vi "USBImageWthFileOutputManual.vi"() -> ()   [LabVIEW 2017]
uses:
  <vilib>/Utility/file.llb/Write Delimited Spreadsheet (I64).vi
  atmcd32d.dll
panel:
  in  "?":bool
  in  "?":bool
  out "Status":u32
  out "Get Status":u32
  out "Vertical Binned Waveform Graph":i32[](graph)
  out "Intensity Graph":i32[][](graph)
  out "Set Image":u32
  out "Set Gate Mode":u32
  out "Shut Down":u32
  out "Detector Y Pixels":i32
  out "Get Detector":u32
  out "Set Exposure Time":u32
  out "Set Trigger Mode":u32
  out "Set Readout Mode":u32
  out "Set Acquisition Mode":u32
  out "Check Timings":u32
  out "Detector X Pixels":i32
  out "Start Acquisition":u32
  out "Get Acquired Data":u32
  out "Calculated Exposure Value":sgl format="%.5f"
  in  "Exposure Time (secs)":sgl format="%.2f"
  out "Initialize":u32
  in  "Trigger":u32(ring) items=["Internal", "External"]
  # "Status"
  # "Return values"
  # "USB iStarIMAG32at.VI"
  # "Acquisition Mode: Single Scan\nReadout Mode: Full Resolution Image"
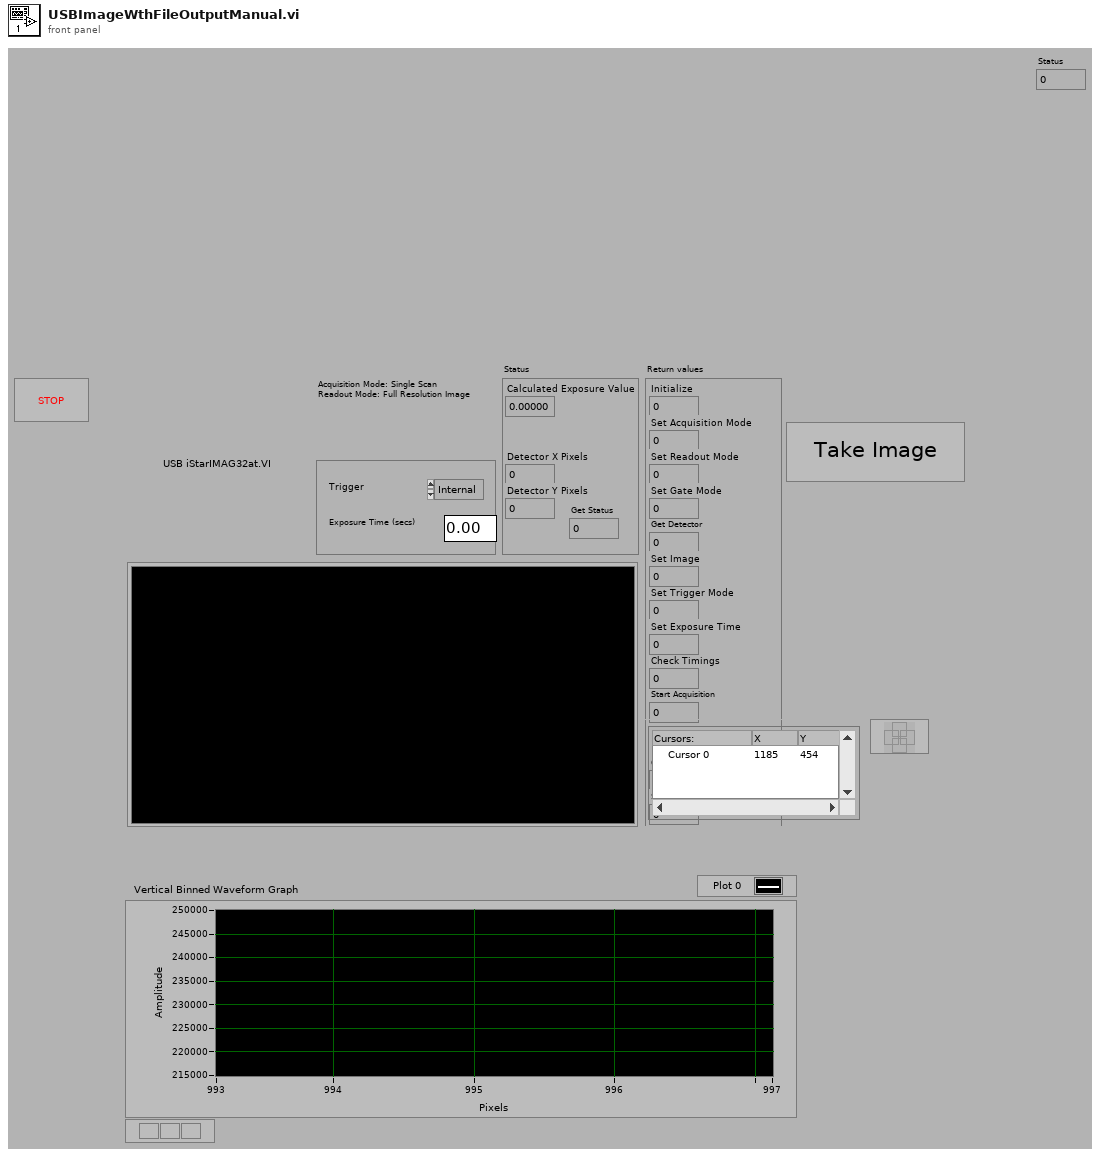
[diagram p1: front panel]
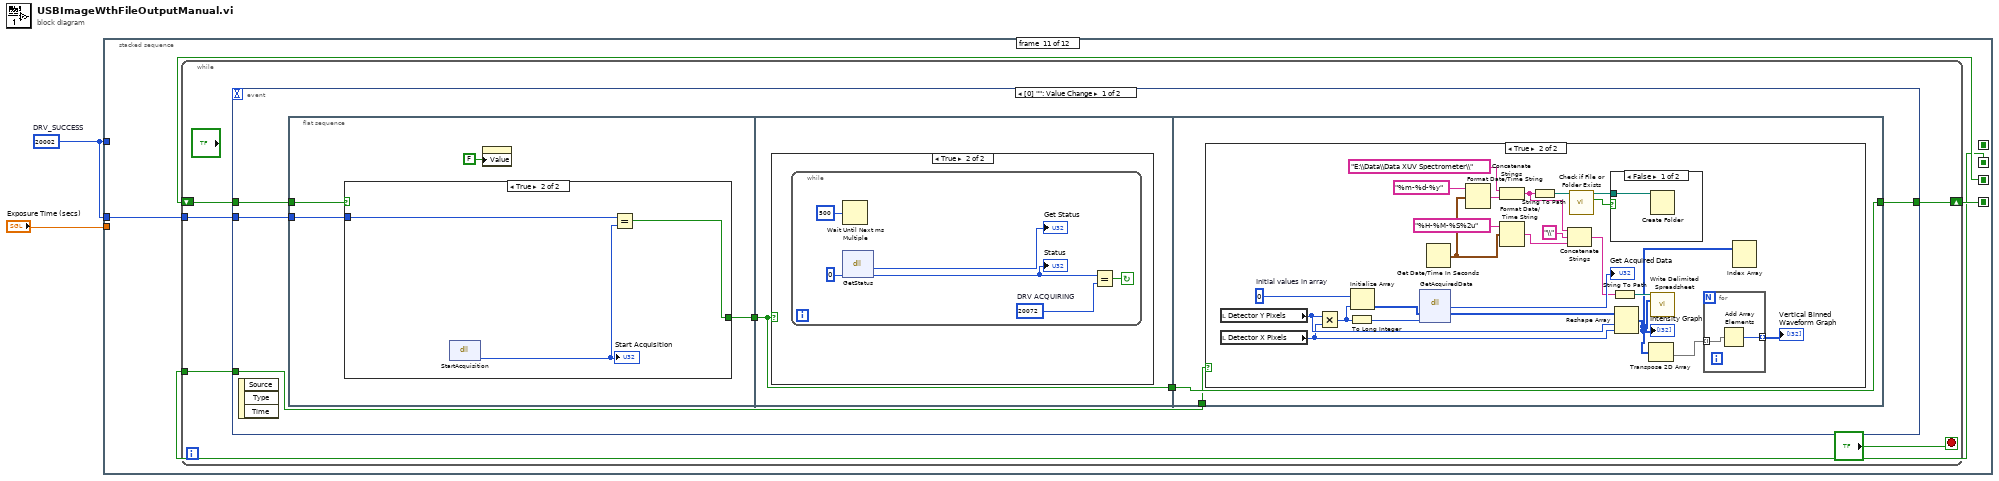
[diagram p0: block diagram]
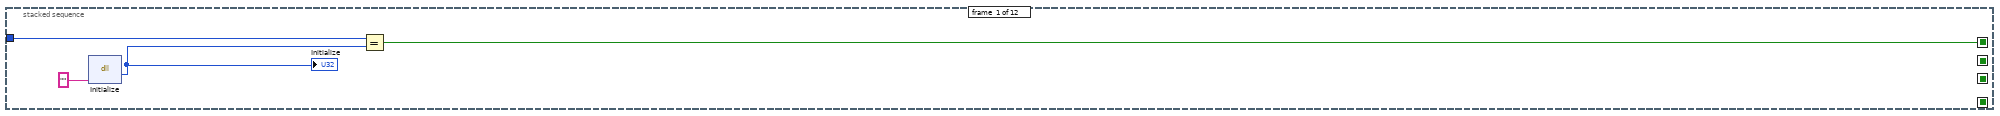
[diagram p2: hidden frame]
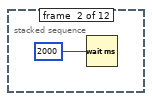
[diagram p3: hidden frame]
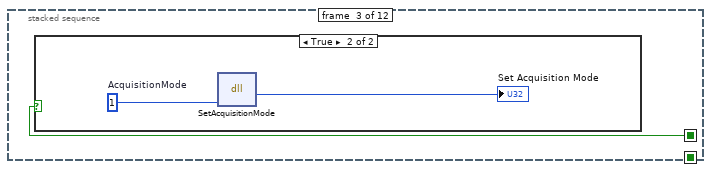
[diagram p4: hidden frame]
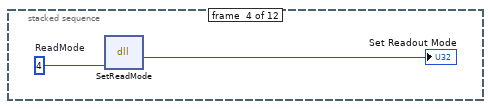
[diagram p6: hidden frame]
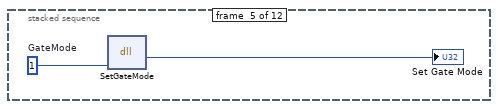
[diagram p7: hidden frame]
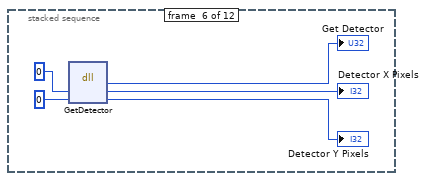
[diagram p8: hidden frame]
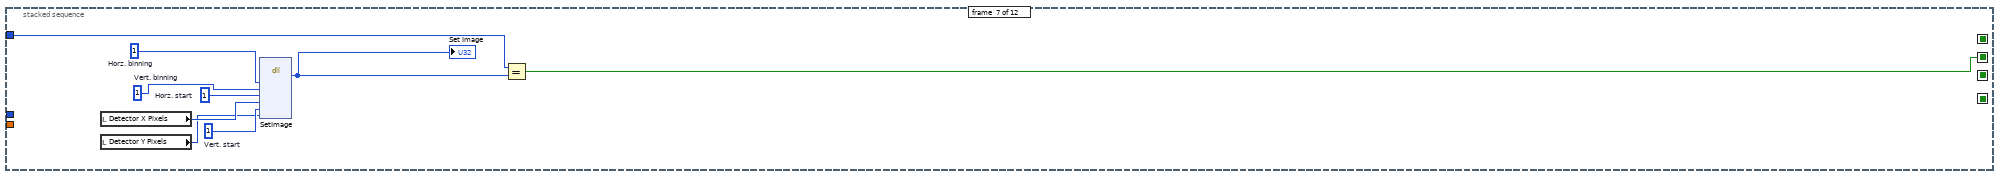
[diagram p9: hidden frame]
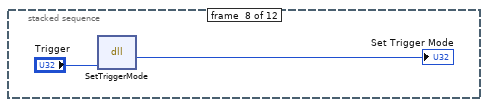
[diagram p10: hidden frame]
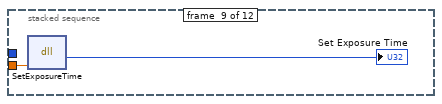
[diagram p11: hidden frame]
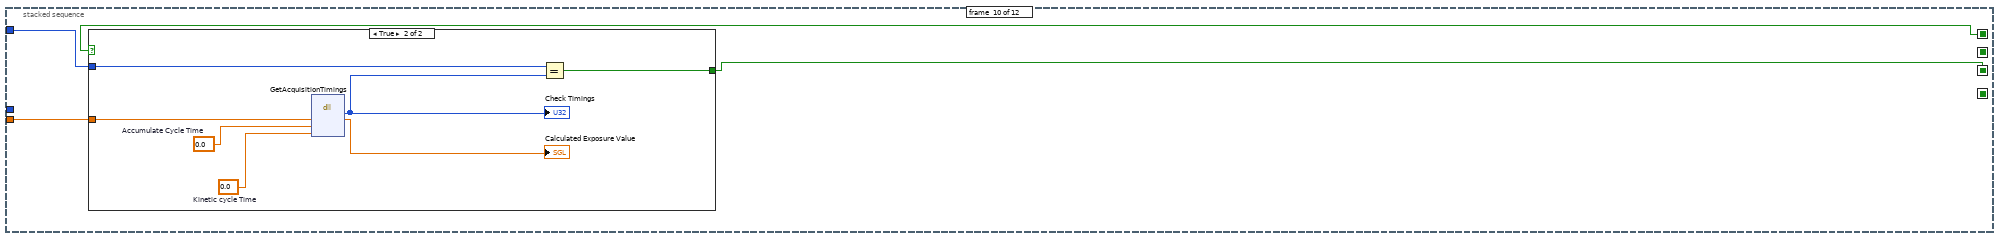
[diagram p12: hidden frame]
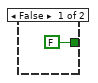
[diagram p13: hidden frame]
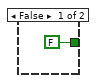
[diagram p14: hidden frame]
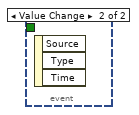
[diagram p18: hidden frame]
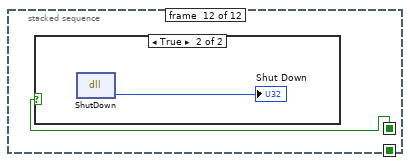
[diagram p19: hidden frame]
diagram:
  w1 = 20002  # DRV_SUCCESS
  n1 = stacked-sequence {
    seq-local: [w4 _ _ _ _ _ _ _ _ _ _ _] -> [_ _ w8 _ _ _ _ _ _ w33 _ w104]
    seq-local: [_ _ _ _ _ _ _ _ _ w34 _ _] -> [_ _ _ _ _ _ _ _ _ _ w48 _]
    seq-local: [_ _ _ _ _ _ _ _ _ _ w46 _] -> [_ _ _ _ _ _ _ _ _ _ _ _]
    seq-local: [_ _ _ _ _ _ w20 _ _ _ _ _] -> [_ _ _ _ _ _ _ _ _ _ w45 _]
    tunnel: "Exposure Time (secs)" -> [_ _ _ _ _ _ _ _ w32 w36 _ _]
    tunnel: w1 -> [w5 _ _ _ _ _ w22 _ _ w35 _ _]
    tunnel: w1 -> [_ _ _ _ _ _ _ _ _ _ w47 _]
    frame #0 {
      n2 = dll-call lib="atmcd32d.dll" fn="Initialize" label="Call Library Function Initialize"("") -> (w6:u32)  [unwired: 4 in, 2 out]
      "Initialize" <- w6
      n3 = Equal?(x=w5, y=w6) -> (x = y?=w4:bool)
    }
    frame #1 {
      n4 = Wait (ms)(milliseconds to wait=u32 2000) -> ()  [unwired: 1 out]
    }
    frame #2 {
      n5 = case shown="True" w8 {
        frame False {
        }
        frame True {
          w10 = u16 1  # AcquisitionMode
          n6 = dll-call lib="atmcd32d.dll" fn="SetAcquisitionMode" label="Call Library Function SetAcquisitionMode"(w10) -> (→"Set Acquisition Mode":u32)  [unwired: 4 in, 2 out]
        }
      }
    }
    frame #3 {
      w12 = u16 4  # ReadMode
      n7 = dll-call lib="atmcd32d.dll" fn="SetReadMode" label="Call Library Function SetReadMode"(w12) -> (→"Set Readout Mode":u32)  [unwired: 4 in, 2 out]
    }
    frame #4 {
      w14 = u16 1  # GateMode
      n8 = dll-call lib="atmcd32d.dll" fn="SetGateMode" label="Call Library Function SetGateMode"(w14) -> (→"Set Gate Mode":u32)  [unwired: 4 in, 2 out]
    }
    frame #5 {
      n9 = dll-call lib="atmcd32d.dll" fn="GetDetector" label="Call Library FunctionGetDetector"(i16 0, i16 0) -> (→"Get Detector":u32, →"Detector X Pixels":i32, →"Detector Y Pixels":i32)  [unwired: 3 in, 2 out]
    }
    frame #6 {
      w25 = u16 1  # Vert. start
      w26 = u16 1  # Horz. start
      w27 = u16 1  # Vert. binning
      w28 = u16 1  # Horz. binning
      n10 = local read "Detector X Pixels"() -> (w24:i32)
      n11 = local read "Detector Y Pixels"() -> (w23:i32)
      n12 = dll-call lib="atmcd32d.dll" fn="SetImage" label="Call Library Function SetImage"(w28, w27, w26, w24, w25, w23) -> (w21:u32)  [unwired: 9 in, 2 out]
      "Set Image" <- w21
      n13 = Equal?(x=w22, y=w21) -> (x = y?=w20:bool)
    }
    frame #7 {
      n14 = dll-call lib="atmcd32d.dll" fn="SetTriggerMode" label="Call Library Function SetTrigger Mode"("Trigger") -> (→"Set Trigger Mode":u32)  [unwired: 4 in, 2 out]
    }
    frame #8 {
      n15 = dll-call lib="atmcd32d.dll" fn="SetExposureTime" label="Call Library FunctionSet Exposure Time"(w32) -> (→"Set Exposure Time":u32)  [unwired: 4 in, 2 out]
    }
    frame #9 {
      n16 = case shown="True" w33 {
        tunnel: w36 -> [_ w41]
        tunnel: w35 -> [_ w38]
        tunnel: [FALSE w40] -> w34
        frame False {
        }
        frame True {
          w43 = sgl 0.0  # Accumulate Cycle Time
          w44 = sgl 0.0  # Kinetic cycle Time
          n17 = dll-call lib="atmcd32d.dll" fn="GetAcquisitionTimings" label="Call Library Function Check Timings"(w41, w43, w44) -> (w39:u32, →"Calculated Exposure Value":sgl)  [unwired: 5 in, 2 out]
          "Check Timings" <- w39
          n18 = Equal?(x=w38, y=w39) -> (x = y?=w40:bool)
        }
      }
    }
    frame #10 {
      n19 = while {
        tunnel: w47 -> [w52]
        tunnel: w45 -> [w50]
        shift-right: [w51] -> w46
        shift-left: w48 -> [w53]
        stop <- "?" stop-if-true
        n20 = event shown="[0] \"\": Value Change" {
          selector: _ -> [_ _]
          dyn-events: _ -> [_ _]
          timeout: _ -> [_ _]
          tunnel: w53 -> [w57 _]
          tunnel: w52 -> [w56 _]
          tunnel: [w55 _] -> w51
          tunnel: w50 -> [w54 _]
          event Value Change {
            n21 = event-data() -> ()  [unwired: 1 in, 3 out]
            n22 = flat-sequence {
              tunnel: w57 -> [w63]
              tunnel: w56 -> [w62]
              tunnel: [w61] -> w59
              tunnel: w59 -> [w68]
              tunnel: [w68] -> w58
              tunnel: [w76] -> w55
              tunnel: w58 -> [w76]
              tunnel: w54 -> [w75]
              frame #0 {
                n23 = case shown="True" w63 {
                  tunnel: [FALSE w66] -> w61
                  tunnel: w62 -> [_ w65]
                  frame False {
                  }
                  frame True {
                    n24 = dll-call lib="atmcd32d.dll" fn="StartAcquisition" label="Call Library Function start acquisition"() -> (w67:u32)  [unwired: 3 in, 2 out]
                    "Start Acquisition" <- w67
                    n25 = Equal?(x=w65, y=w67) -> (x = y?=w66:bool)
                  }
                }
                n26 = property class="Bool (strict)"("Value"=FALSE ("Take image")) -> ()  [unwired: 2 in, 2 out]
              }
              frame #1 {
                n27 = case shown="True" w68 {
                  frame False {
                  }
                  frame True {
                    n28 = while {
                      stop <- w72 continue-if-true
                      w71 = u16 20072  # DRV ACQUIRING
                      n29 = Wait Until Next ms Multiple(millisecond multiple=u32 500) -> ()  [unwired: 1 out]
                      n30 = dll-call lib="atmcd32d.dll" fn="GetStatus" label="Call Library Function GetAcquisitionStatus"(u16 0) -> (→"Get Status":u32, w70:u32)  [unwired: 3 in, 2 out]
                      "Status" <- w70
                      n31 = Equal?(x=w70, y=w71) -> (x = y?=w72:bool)
                    }
                  }
                }
              }
              frame #2 {
                n32 = case shown="True" w75 {
                  frame False {
                  }
                  frame True {
                    w100 = 0  # Initial values in array
                    n33 = local read "Detector Y Pixels"() -> (w94:i32)
                    n34 = local read "Detector X Pixels"() -> (w93:i32)
                    n35 = Multiply(x=w94, y=w93) -> (x*y=w96:i32)
                    n36 = To Long Integer(number=w96) -> (32bit integer=w97:i32)
                    n37 = Initialize Array "Initialize Array"(w100, w96) -> (w98:i32[])
                    n38 = dll-call lib="atmcd32d.dll" fn="GetAcquiredData" label="Call Library Function Get Acquired data"(w98, w97) -> (→"Get Acquired Data":u32, w95:i32[])  [unwired: 4 in, 2 out]
                    n39 = Get Date/Time In Seconds() -> (seconds since 1Jan1904=w90:timestamp)
                    n40 = Format Date/Time String(time format string (%c)="%m-%d-%y", seconds (now)=w90) -> (date/time string=w88:string)  [unwired: 1 in]
                    n41 = Concatenate Strings("E:\\Data\\Data XUV Spectrometer\\" ("string"), w88) -> (w91:string)
                    n42 = Format Date/Time String(time format string (%c)="%H-%M-%S%2u", seconds (now)=w90) -> (date/time string=w89:string)  [unwired: 1 in]
                    n43 = String To Path(string=w91) -> (path=w87:path)
                    n44 = Concatenate Strings(w91, "\\" ("string"), w89) -> (w92:string)
                    n45 = call <vilib>:"Check if File or Folder Exists.vi"("path"=w87) -> ("file or folder exists?"=w85:bool, "dup path"=w86:path)  [unwired: 8 in, 1 out]
                    n46 = case shown="False" w85 {
                      tunnel: w86 -> [w103 _]
                      frame False {
                        n47 = Create Folder(path (use dialog)=w103) -> ()  [unwired: 2 in, 3 out]
                      }
                      frame True {
                      }
                    }
                    n48 = String To Path(string=w92) -> (path=w80:path)
                    n49 = Reshape Array(w95, w94, w93) -> (w78:i32[][])
                    "Intensity Graph" <- w78
                    n50 = Transpose 2D Array(2D array=w78) -> (transposed array=w79:i32[][])
                    n51 = call-poly <vilib>:"Write Delimited Spreadsheet.vi"("file path (dialog if empty)"=w80, "2D data"=w78) -> ()  [unwired: 12 in, 2 out]
                    n52 = for {
                      tunnel: w79 -> [w102] mode=indexing
                      tunnel: [w101] -> w77 mode=indexing
                      n53 = Add Array Elements(numeric array=w102) -> (sum=w101:i32)
                    }
                    "Vertical Binned Waveform Graph" <- w77
                    n54 = Index Array(array=w78) -> ()  [unwired: 2 in, 1 out]
                  }
                }
              }
            }
          }
          event Value Change {
            n55 = event-data() -> ()  [unwired: 1 in, 3 out]
          }
        }
      }
    }
    frame #11 {
      n56 = case shown="True" w104 {
        frame False {
        }
        frame True {
          n57 = dll-call lib="atmcd32d.dll" fn="ShutDown" label="Call Library Function Shutdown"() -> (→"Shut Down":u32)  [unwired: 3 in, 2 out]
        }
      }
    }
  }
